vi "reward_behavior_michelle_visjitter_conswinAdapt_enticefx_TSLogFC2.vi"() -> ()   [LabVIEW 2019]
doc: "The myRIO Project template acquires acceleration data from the onboard accelerometer and displays the changes of acceleration values in a waveform chart."
uses:
  <vilib>/Analysis/Matrix/Datatypes/RealMatrix.ctl
  <vilib>/myRIO/Common/Instrument Driver Framework/myRIO v1.0/Encoder/typedefs/Encoder Signal Mode.ctl
  <vilib>/myRIO/Instrument Drivers/Onboard IO/Encoder/typedefs/Encoder Reference.ctl
  <vilib>/myRIO/Common/Instrument Driver Framework/Utilities/typedefs/myRIO Generic Hardware Reference.ctl
  <vilib>/myRIO/Common/Instrument Driver Framework/Utilities/typedefs/Hardware Version Enum.ctl
  <vilib>/myRIO/Common/Instrument Driver Framework/Utilities/typedefs/myRIO v1.0 Reference.ctl
  <vilib>/myRIO/Common/Instrument Driver Framework/Utilities/typedefs/Generic FPGA Reference.ctl
  <vilib>/myRIO/Common/Instrument Driver Framework/myRIO v1.0/Encoder/typedefs/Encoder Channels Enum.ctl
  <vilib>/myRIO/Common/Instrument Driver Framework/myRIO v1.0/Encoder/typedefs/Encoder Configuration v1.0.ctl
  <vilib>/userdefined/High Color/nirio_resource_hc.ctl
  <vilib>/myRIO/Instrument Drivers/Onboard IO/DIO/typedefs/DIO Reference.ctl
  <vilib>/myRIO/Common/Instrument Driver Framework/myRIO v1.0/DIO/typedefs/DIO Channels List.ctl
  <vilib>/myRIO/Common/Instrument Driver Framework/myRIO v1.0/DIO/typedefs/DIO Channels Enum.ctl
  <vilib>/myRIO/Common/Instrument Driver Framework/Utilities/vis/Is FPGA Ref Available.vi
  <vilib>/myRIO/Common/Instrument Driver Framework/myRIO v1.0/Encoder/vis/myRIO v1.1 Open Encoder.vi
  <vilib>/myRIO/Instrument Drivers/Onboard IO/Encoder/vis/Read.vi
  <vilib>/myRIO/Common/Instrument Driver Framework/myRIO v1.0/DIO/vis/myRIO v1.1 Open DIO.vi
  <vilib>/myRIO/Instrument Drivers/Onboard IO/DIO/vis/Write.vi
  <vilib>/myRIO/Instrument Drivers/Onboard IO/DIO/vis/Read.vi
  <vilib>/myRIO/Common/Instrument Driver Framework/Utilities/vis/Validate Channels.vi
  <vilib>/myRIO/Common/Instrument Driver Framework/myRIO v1.0/Encoder/vis/myRIO v1.0 Reserve Encoder.vi
  <vilib>/myRIO/Common/Instrument Driver Framework/myRIO v1.0/DIO/vis/myRIO v1.0 Reserve DIO.vi
  <vilib>/myRIO/Common/Instrument Driver Framework/myRIO v1.0/Encoder/vis/myRIO v1.0 Build MUX Configuration Encoder.vi
  <vilib>/myRIO/Common/Instrument Driver Framework/myRIO v1.0/Resource Manager/vis/myRIO v1.0 Reserve Channel List.vi
  <vilib>/myRIO/Common/Instrument Driver Framework/myRIO v1.0/DIO/vis/myRIO v1.0 Build MUX Configuration DIO.vi
  <vilib>/myRIO/Common/Instrument Driver Framework/myRIO v1.0/Resource Manager/vis/myRIO v1.0 Create Configuration List.vi
  <vilib>/myRIO/Common/Instrument Driver Framework/myRIO v1.0/Resource Manager/vis/myRIO v1.0 Reserve Channel.vi
  <vilib>/myRIO/Common/Instrument Driver Framework/myRIO v1.0/Resource Manager/vis/myRIO v1.0 Unreserve Channel.vi
  <vilib>/myRIO/Common/Instrument Driver Framework/myRIO v1.0/Resource Manager/vis/myRIO v1.0 Build Mutex Name.vi
  <vilib>/Utility/VariantDataType/GetNumericInfo.vi
  <vilib>/Utility/error.llb/Error Cluster From Error Code.vi
  <vilib>/myRIO/Common/Instrument Driver Framework/myRIO v1.0/myRIO v1.1 Open.vi
  <vilib>/myRIO/Common/Instrument Driver Framework/Utilities/vis/IO Manager.vi
  <vilib>/myRIO/Common/Instrument Driver Framework/Utilities/vis/Configuration Manager.vi
  <vilib>/myRIO/Common/Instrument Driver Framework/myRIO v1.0/Resource Manager/vis/myRIO v1.0 Configure IO.vi
  <vilib>/myRIO/Common/Instrument Driver Framework/myRIO v1.0/myRIO v1.0 Close.vi
  <vilib>/myRIO/Common/Instrument Driver Framework/myRIO v1.0/Encoder/vis/myRIO v1.0 Configure Encoder.vi
  <vilib>/myRIO/Common/Instrument Driver Framework/myRIO v1.0/Encoder/vis/myRIO v1.0 Read Encoder.vi
  <vilib>/myRIO/Common/Instrument Driver Framework/myRIO v1.0/DIO/vis/myRIO v1.0 Read DIO.vi
  <vilib>/myRIO/Common/Instrument Driver Framework/myRIO v1.0/DIO/vis/myRIO v1.0 Write DIO.vi
  <vilib>/myRIO/Express VI/Onboard IO/Encoder/Encoder Express VI.xnode
  <vilib>/myRIO/Instrument Drivers/Onboard IO/Encoder/vis/myRIO Encoder Open.xnode
  <vilib>/myRIO/Express VI/Onboard IO/DI/DI Express VI.xnode
  <vilib>/myRIO/Instrument Drivers/Onboard IO/DIO/vis/myRIO DIO Open.xnode
  <vilib>/myRIO/Express VI/Onboard IO/DO/DO Express VI.xnode
  <vilib>/myRIO/Instrument Drivers/Onboard IO/Encoder/Encoder.lvlib
  <vilib>/myRIO/Instrument Drivers/Onboard IO/DIO/DIO.lvlib
  <vilib>/Analysis/Matrix/NI_Matrix.lvlib
panel:
  out "EntTS":dbl[][](array[numeric])
  out "TimeLag":dbl
  out "Lag2":dbl
  out "TestTime":dbl
  out "RewTS":dbl[][](array[numeric])
  out "ConsTS":dbl[][](array[numeric])
  out "LickTS":dbl[][](array[numeric])
  out "ContrastChoice":dbl
  out "Its":i32
  out "BurstCriteria":dbl
  out "LickBurst 2":bool
  out "LickBurst":bool
  out "Enticements":i32
  in  "Entice":bool
  out "Misses":i32
  out "GoAhead":bool
  out "TimeOutDuration":i32
  out "ActiveTime":dbl
  out "ConsumptionGo":bool=TRUE
  out "Consumption_Period":i32
  out "Watch_Display":bool=TRUE
  in  "Give reward":bool
  out "Timings":dbl[](array[numeric])
  out "ISI":dbl
  out "ISI start time":dbl
  out "Time_out":bool=TRUE
  out "Time since lick":dbl
  out "Time of last lick":dbl
  out "Rewarded trials":dbl[](array[numeric])
  out "Rewards":u16
  out "Active Trial":bool
  out "Array temp2":T1
  out "Stimuli Loaded":bool
  out "Stim_ID":dbl[](array[numeric])
  out "Reward_mat":dbl[](array[numeric])
  out "Reward":bool=TRUE
  out "Frame clock":i32
  out "Licks":u32
  out "Lick":bool
  out "Time":dbl
  out "Stop":bool
  in  "Frames to collect":u32
  out "Overflow?":bool
  out "Counter Value":i32
  out "Velocity":dbl
  out "Velocity Plot":dbl[](graph)
  out "Velocity array":dbl[](array[numeric])
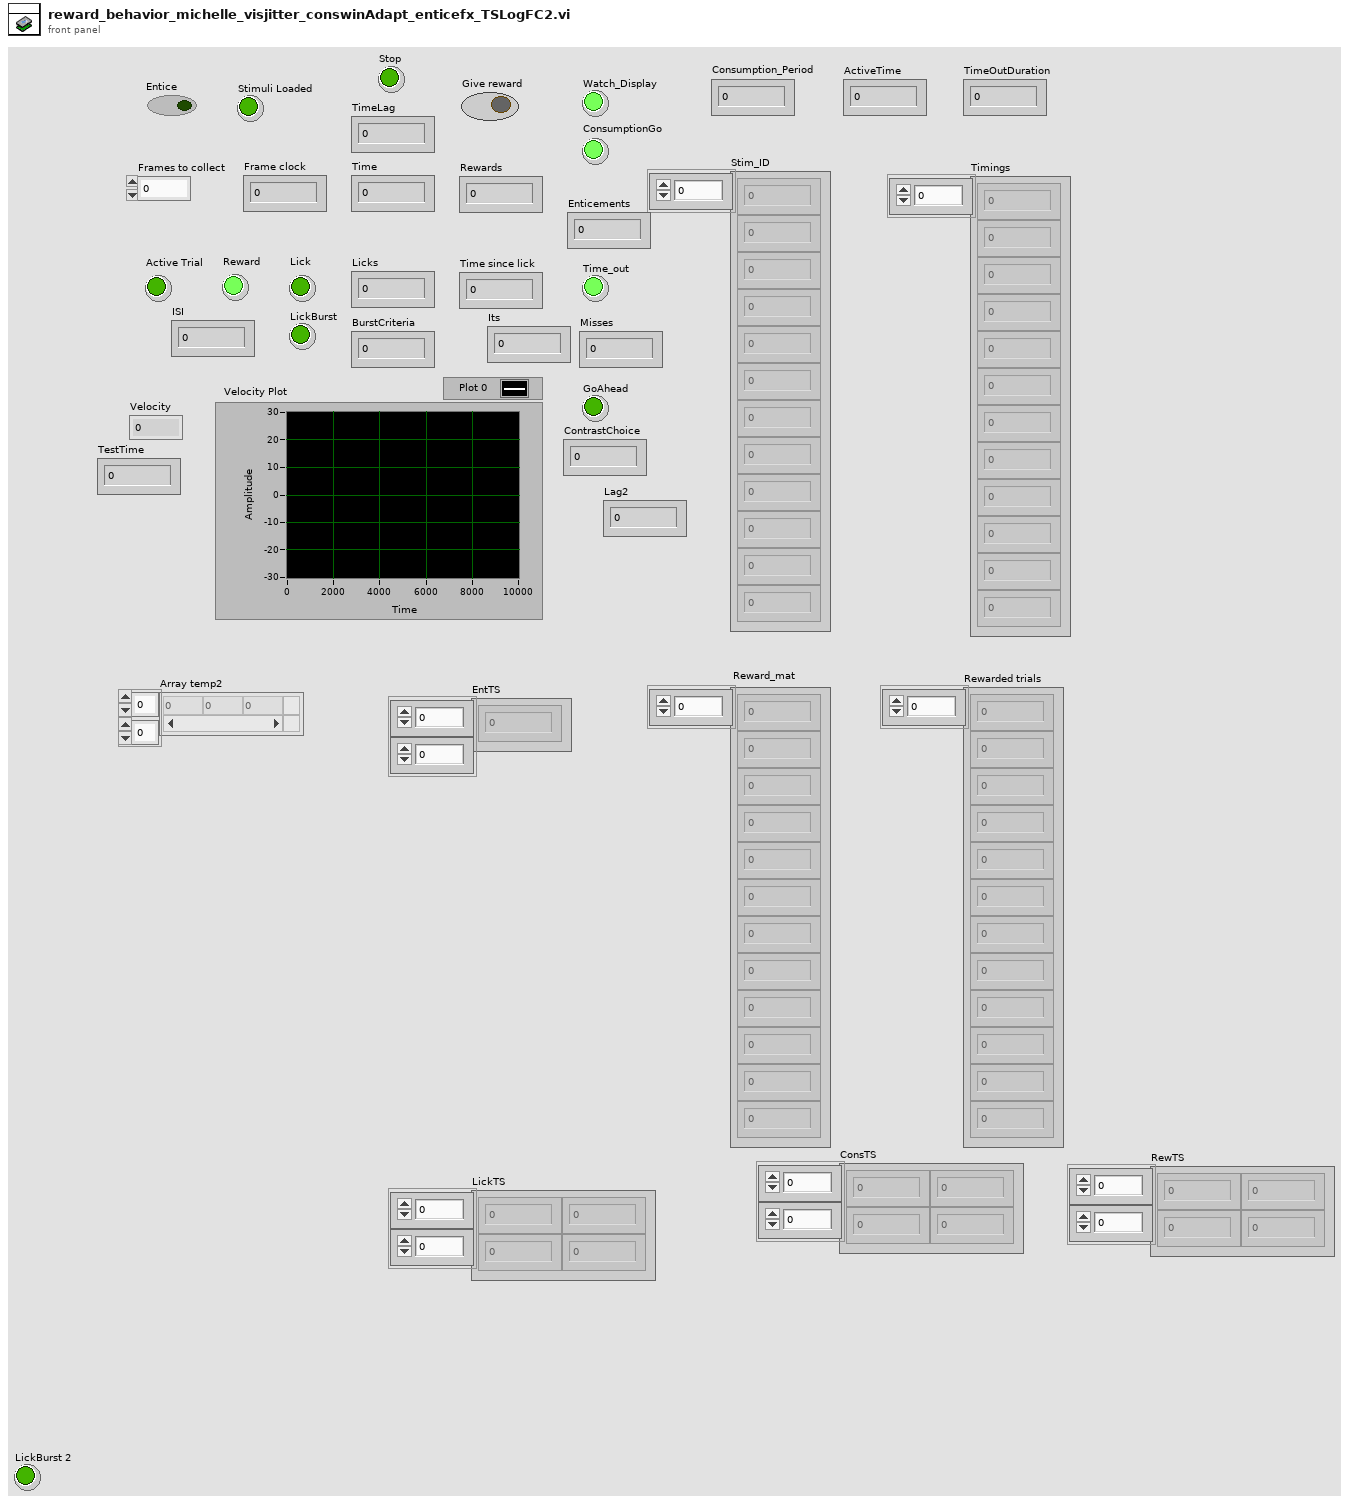
[diagram p1: front panel]
types:
  T1 = typedef "NI_Matrix.lvlib/RealMatrix.ctl" = dbl[][]
  T2 = typedef "Encoder.lvlib/Encoder Reference.ctl" = cluster{"myRIO Reference":T3, "Encoder Channels Enum":T7}
  T3 = typedef "myRIO Generic Hardware Reference.ctl" = cluster{"myRIO Model":T4, "myRIO Hardware Reference":T5}
  T4 = typedef "Hardware Version Enum.ctl" = enum16{"Unknown", "myRIO-1900", "myRIO-1950", "roboRIO", "NI ELVIS RIO CM", "ELVIS III"}
  T5 = typedef "myRIO v1.0 Reference.ctl" = cluster{"Generic FPGA Reference":T6, "Allow multiple opens":bool}
  T6 = typedef "Generic FPGA Reference.ctl" = refnum<k20>
  T7 = typedef "Encoder Channels Enum.ctl" = enum16{"Not Connected", "C/ENC0", "C/ENC1", "A/ENC", "A/ENC0", "A/ENC1", "A/ENC2", "A/ENC3", "A/ENC4", "A/ENC5", "A/ENC6", "A/ENC7", "A/ENC8", "A/ENC9", "B/ENC", "B/ENC0", "B/ENC1", "B/ENC2", "B/ENC3", "B/ENC4", "B/ENC5", "B/ENC6", "B/ENC7", "B/ENC8", "B/ENC9", "DIO/ENC0", "DIO/ENC1", "DIO/ENC2", "DIO/ENC3", "DIO/ENC4"}
  T8 = typedef "Encoder Signal Mode.ctl" = enum16{"Quadrature phase signal", "Step and direction signal"}
  T9 = typedef "nirio_resource_hc.ctl" = tag
  T10 = typedef "DIO.lvlib/DIO Reference.ctl" = cluster{"myRIO Reference":T3, "DIO Channels List":T11}
  T11 = typedef "DIO Channels List.ctl" = T12[]
  T12 = typedef "DIO Channels Enum.ctl" = enum16{"Not Connected", "C/DIO0", "C/DIO1", "C/DIO2", "C/DIO3", "C/DIO4", "C/DIO5", "C/DIO6", "C/DIO7", "A/DIO0", "A/DIO1", "A/DIO2", "A/DIO3", "A/DIO4", "A/DIO5", "A/DIO6", "A/DIO7", "A/DIO8", "A/DIO9", "A/DIO10", "A/DIO11", "A/DIO12", "A/DIO13", "A/DIO14", "A/DIO15", "A/DIO16", "A/DIO17", "A/DIO18", "A/DIO19", "B/DIO0", "B/DIO1", "B/DIO2", "B/DIO3", "B/DIO4", "B/DIO5", "B/DIO6", "B/DIO7", "B/DIO8", "B/DIO9", "B/DIO10", "B/DIO11", "B/DIO12", "B/DIO13", "B/DIO14", "B/DIO15", "B/DIO16", "B/DIO17", "B/DIO18", "B/DIO19", "LED0", "LED1", "LED2", "LED3", "Button0", "DIO/DIO0", "DIO/DIO1", "DIO/DIO2", "DIO/DIO3", "DIO/DIO4", "DIO/DIO5", "DIO/DIO6", "DIO/DIO7", "DIO/DIO8", "DIO/DIO9", "SPI/CS0", "SPI/CS1", "SPI/CS2", "SPI/CS3", "LED RADIO (Green)", "LED RADIO (Red)", "LED COMM (Green)", "LED COMM (Red)", "LED MODE (Green)", "LED MODE (Red)"}
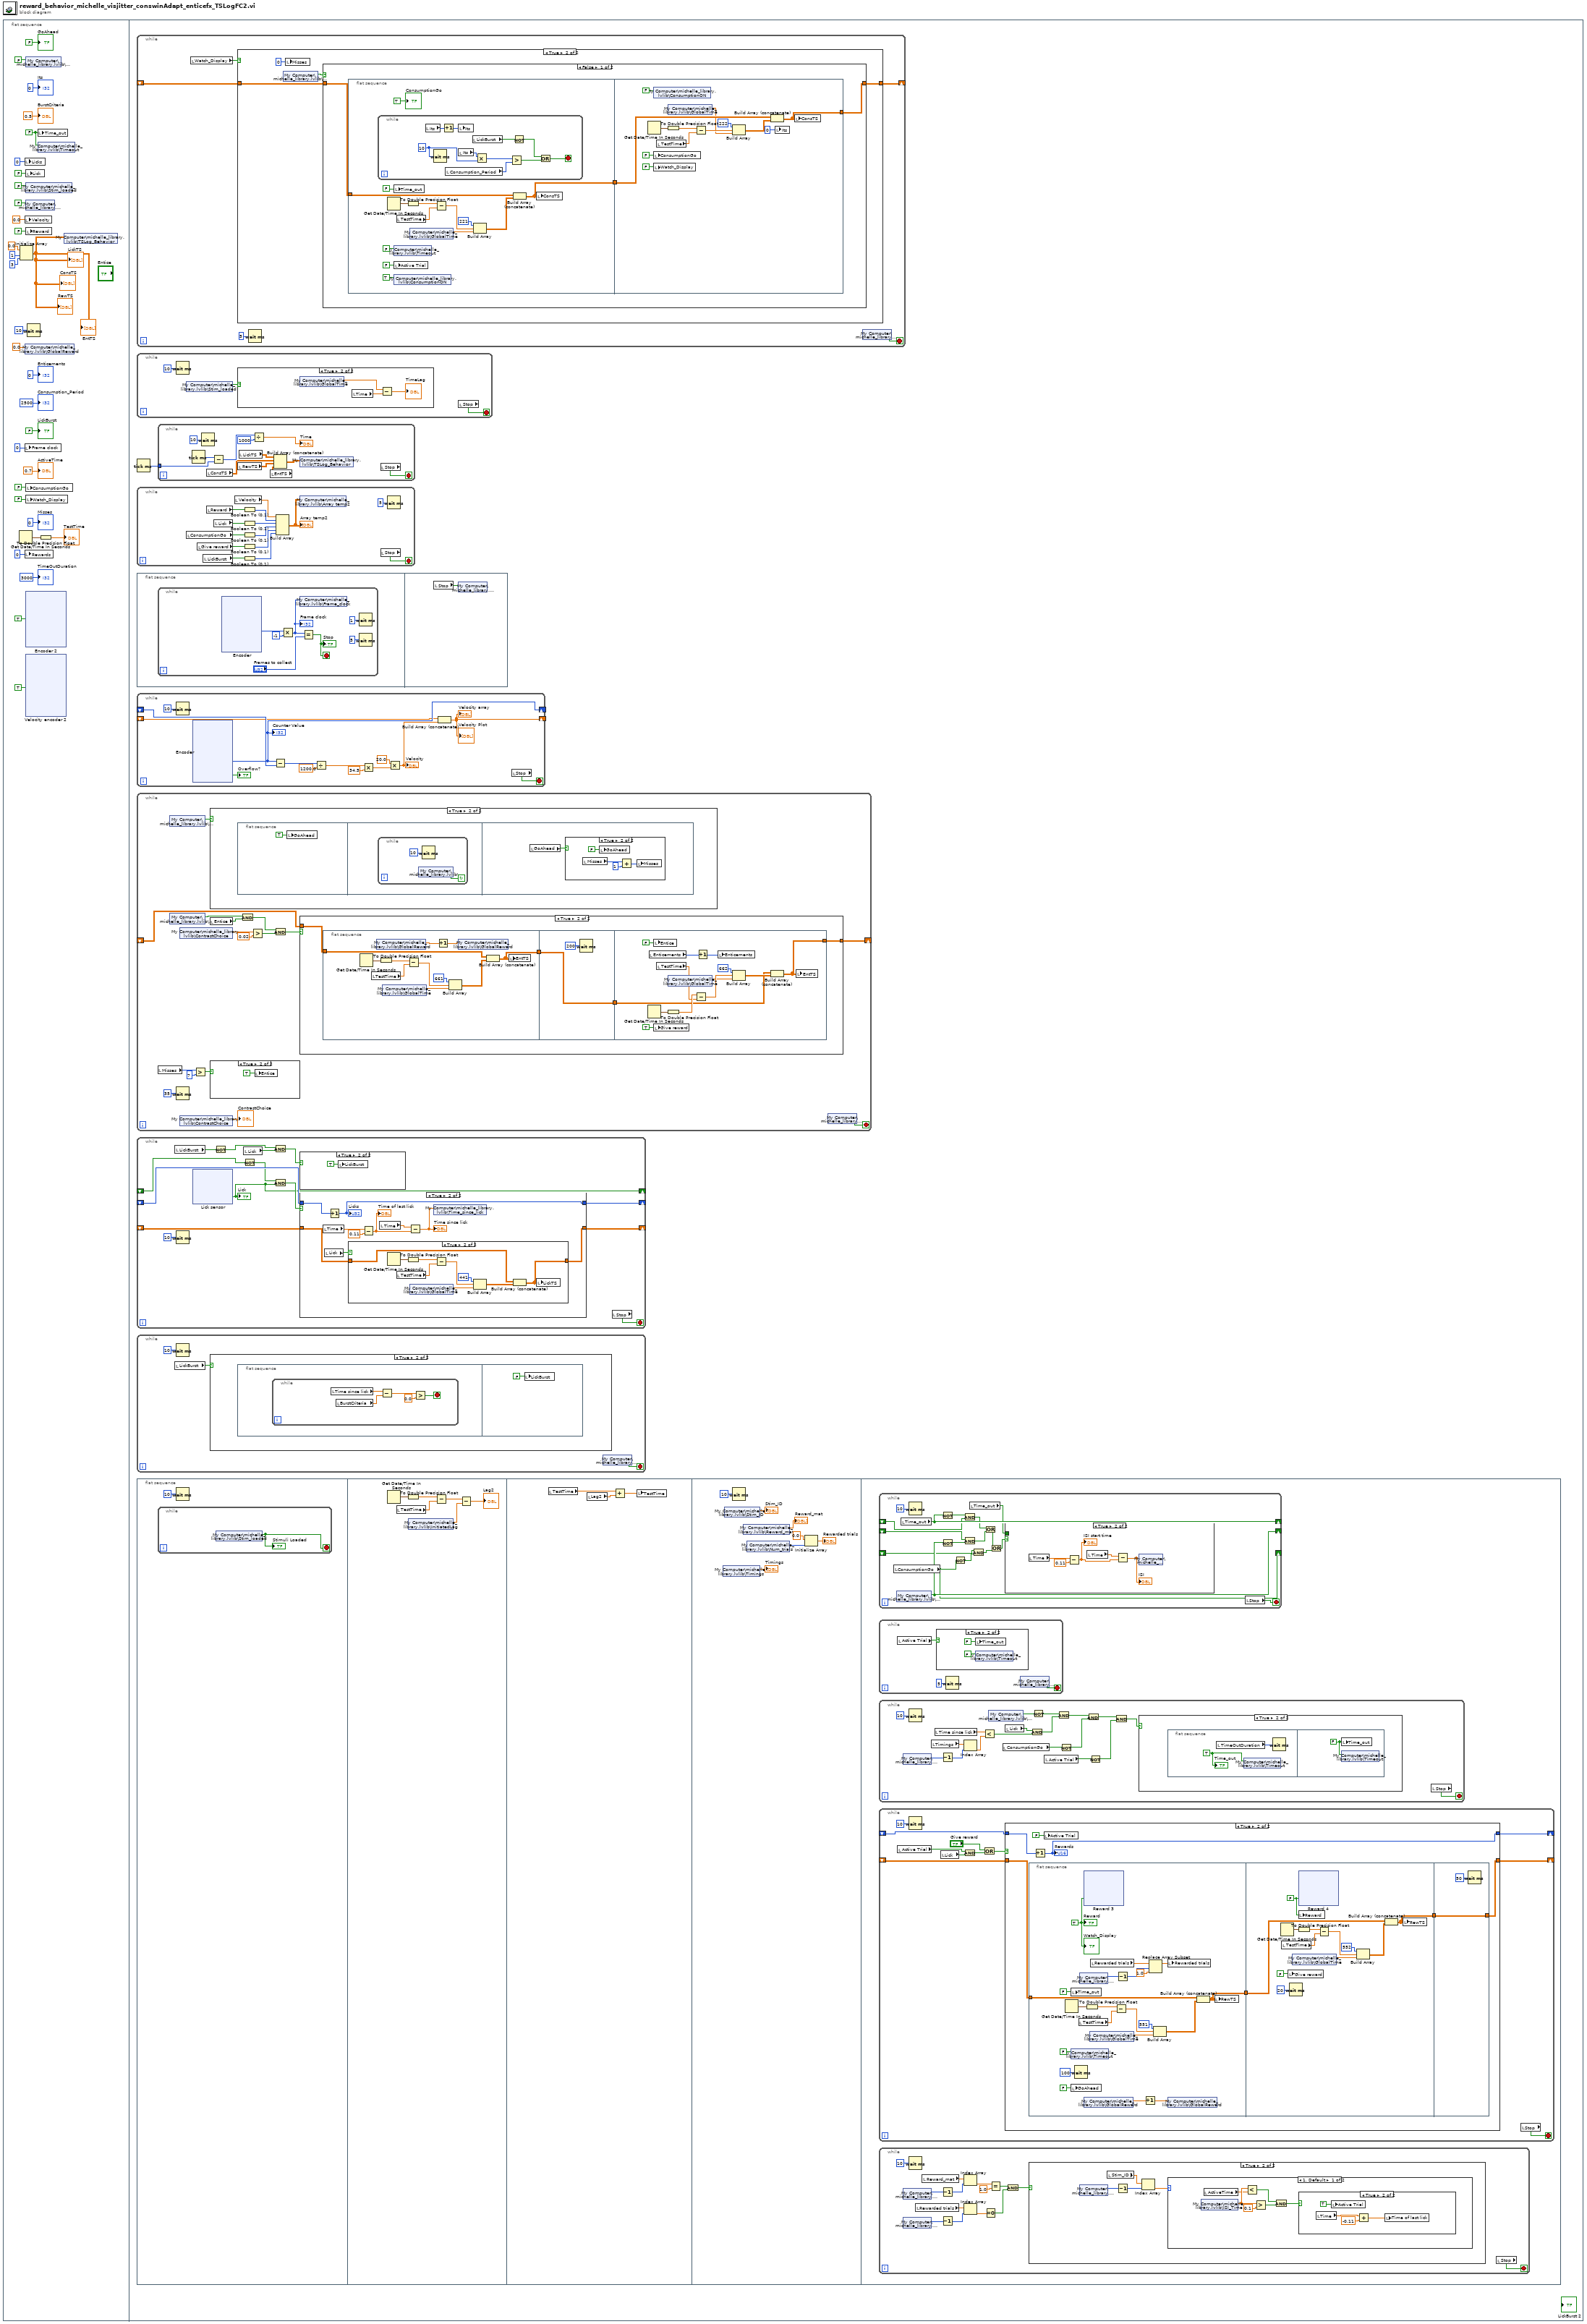
[diagram p0: block diagram]
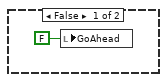
[diagram p6: hidden frame]
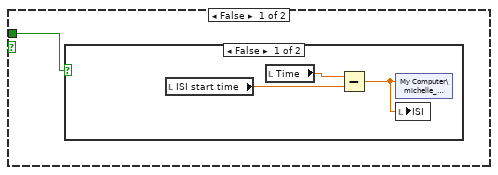
[diagram p12: hidden frame]
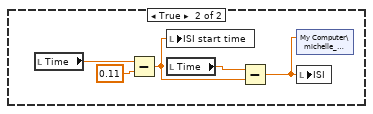
[diagram p13: hidden frame]
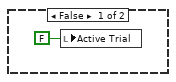
[diagram p14: hidden frame]
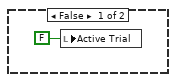
[diagram p15: hidden frame]
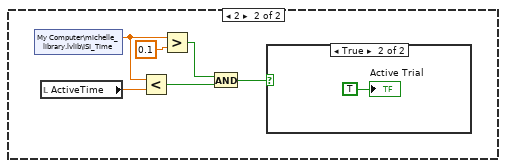
[diagram p16: hidden frame]
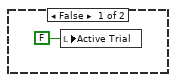
[diagram p17: hidden frame]
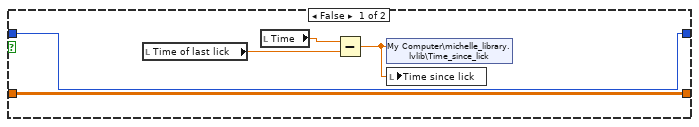
[diagram p20: hidden frame]
diagram:
  n1 = flat-sequence {
    frame #0 {
      w19 = FALSE ("Time_out")
      n2 = Get Date/Time In Seconds() -> (seconds since 1Jan1904=w3:timestamp)
      n3 = Initialize Array(0.0, 1, 3) -> (w1:dbl[][])
      "LickTS" <- w1
      "ConsTS" <- w1
      "RewTS" <- w1
      "EntTS" <- w1
      n4 = local write "Licks"(u32 0 ("Licks")) -> ()
      n5 = local write "Velocity"(0.0 ("Velocity")) -> ()
      n6 = shared-variable "My Computer\\michelle_library.lvlib\\GlobalReward"(0.0) -> ()  [unwired: 1 in, 1 out]
      n7 = local write "Frame clock"(u32 0 ("Frames")) -> ()
      n8 = local write "Rewards"(u16 0 ("Rewards")) -> ()
      n9 = shared-variable "My Computer\\michelle_library.lvlib\\Display"(FALSE ("Display")) -> ()  [unwired: 1 in, 1 out]
      n10 = local write "Lick"(FALSE ("Lick")) -> ()
      n11 = shared-variable "My Computer\\michelle_library.lvlib\\Stim_loaded"(FALSE ("Stim_loaded")) -> ()  [unwired: 1 in, 1 out]
      n12 = shared-variable "My Computer\\michelle_library.lvlib\\Stop"(FALSE ("Stop")) -> ()  [unwired: 1 in, 1 out]
      n13 = local write "Reward"(FALSE ("Give reward")) -> ()
      n14 = local write "ConsumptionGo"(FALSE ("ConsumptionGo")) -> ()
      n15 = local write "Watch_Display"(FALSE ("Watch_Display")) -> ()
      n16 = xnode "Encoder 2"("Reset Counter"=TRUE) -> ()  [unwired: 1 in, 4 out]
      n17 = xnode "Velocity encoder 2"("Reset Counter"=TRUE) -> ()  [unwired: 1 in, 4 out]
      n18 = Wait (ms)(milliseconds to wait=u32 10) -> ()  [unwired: 1 out]
      n19 = local write "Time_out"(w19) -> ()
      n20 = shared-variable "My Computer\\michelle_library.lvlib\\Timeout"(w19) -> ()  [unwired: 1 in, 1 out]
      n21 = To Double Precision Float(number=w3) -> (double precision float=→"TestTime":dbl)
      n22 = shared-variable "My Computer\\michelle_library.lvlib\\TSLog_Behavior"(w1) -> ()  [unwired: 1 in, 1 out]
      "Consumption_Period" <- 2500
      "ActiveTime" <- 0.7
      "TimeOutDuration" <- 3000
      "GoAhead" <- FALSE
      "Misses" <- 0
      "Enticements" <- 0
      "LickBurst" <- FALSE
      "BurstCriteria" <- 0.5
      "Its" <- 0
    }
    frame #1 {
      n23 = while {
        shift-right: [w197] -> _
        shift-left: _ -> [w198]
        stop <- w201 stop-if-true
        n24 = local read "Watch_Display"() -> (w200:bool)
        n25 = case shown="True" w200 {
          tunnel: w198 -> [w202 w204]
          tunnel: [w202 w203] -> w197
          frame False {
          }
          frame True {
            n26 = shared-variable "My Computer\\michelle_library.lvlib\\Display"() -> (w206:bool)  [unwired: 1 in, 1 out]
            n27 = local write "Misses"(0) -> ()
            n28 = case shown="False" w206 {
              tunnel: w204 -> [w209 w247]
              tunnel: [w207 w247] -> w203
              frame False {
                n29 = flat-sequence {
                  tunnel: w209 -> [w212]
                  tunnel: [w211] -> w208
                  tunnel: w208 -> [w237]
                  tunnel: [w236] -> w207
                  frame #0 {
                    n30 = while {
                      stop <- w227 stop-if-true
                      w228 = 10
                      n31 = local read "Its"() -> (w232:i32)
                      n32 = Wait (ms)(milliseconds to wait=w228) -> ()  [unwired: 1 out]
                      n33 = Increment(x=w232) -> (x+1=w231:i32)
                      n34 = local read "Consumption_Period"() -> (w225:i32)
                      n35 = local write "Its"(w231) -> ()
                      n36 = local read "Its"() -> (w229:i32)
                      n37 = local read "LickBurst"() -> (w233:bool)
                      n38 = Multiply(x=w229, y=w228) -> (x*y=w226:i32)
                      n39 = Greater?(x=w226, y=w225) -> (0:w224:bool)
                      n40 = Not(x=w233) -> (.not. x?=w230:bool)
                      n41 = Or(x=w230, y=w224) -> (x .or. y?=w227:bool)
                    }
                    n42 = Get Date/Time In Seconds() -> (seconds since 1Jan1904=w217:timestamp)
                    n43 = local write "Time_out"(FALSE) -> ()
                    n44 = shared-variable "My Computer\\michelle_library.lvlib\\Timeout"(FALSE) -> ()  [unwired: 1 in, 1 out]
                    n45 = local write "Active Trial"(FALSE) -> ()
                    n46 = shared-variable "My Computer\\michelle_library.lvlib\\ConsumptionON"(TRUE) -> ()  [unwired: 1 in, 1 out]
                    n47 = local read "TestTime"() -> (w214:dbl)
                    n48 = To Double Precision Float(number=w217) -> (double precision float=w215:dbl)
                    n49 = shared-variable "My Computer\\michelle_library.lvlib\\GlobalTime"() -> (w210:dbl)  [unwired: 1 in, 1 out]
                    n50 = Subtract(x=w215, y=w214) -> (x-y=w218:dbl)
                    n51 = Build Array(221, w218, w210) -> (w213:T1)
                    n52 = Build Array (concatenate) ("Build Matrix")(w212, w213) -> (w211:T1)
                    n53 = local write "ConsTS"(w211) -> ()
                    "ConsumptionGo" <- TRUE
                  }
                  frame #1 {
                    n54 = Get Date/Time In Seconds() -> (seconds since 1Jan1904=w241:timestamp)
                    n55 = shared-variable "My Computer\\michelle_library.lvlib\\ConsumptionON"(FALSE) -> ()  [unwired: 1 in, 1 out]
                    n56 = local write "ConsumptionGo"(FALSE ("ConsumptionGo")) -> ()
                    n57 = local write "Watch_Display"(FALSE ("Watch_Display")) -> ()
                    n58 = local read "TestTime"() -> (w238:dbl)
                    n59 = To Double Precision Float(number=w241) -> (double precision float=w239:dbl)
                    n60 = shared-variable "My Computer\\michelle_library.lvlib\\GlobalTime"() -> (w234:dbl)  [unwired: 1 in, 1 out]
                    n61 = Subtract(x=w239, y=w238) -> (x-y=w242:dbl)
                    n62 = Build Array(222, w242, w234) -> (w235:T1)
                    n63 = Build Array (concatenate) ("Build Matrix")(w237, w235) -> (w236:T1)
                    n64 = local write "Its"(0) -> ()
                    n65 = local write "ConsTS"(w236) -> ()
                  }
                }
              }
              frame True {
              }
            }
          }
        }
        n66 = Wait (ms)(milliseconds to wait=u32 5) -> ()  [unwired: 1 out]
        n67 = shared-variable "My Computer\\michelle_library.lvlib\\Stop"() -> (w201:bool)  [unwired: 1 in, 1 out]
      }
      n68 = while {
        stop <- w126 stop-if-true
        n69 = Wait (ms)(milliseconds to wait=u32 10) -> ()  [unwired: 1 out]
        n70 = shared-variable "My Computer\\michelle_library.lvlib\\Stim_loaded"() -> (w127:bool)  [unwired: 1 in, 1 out]
        n71 = case shown="True" w127 {
          frame False {
          }
          frame True {
            n72 = shared-variable "My Computer\\michelle_library.lvlib\\GlobalTime"() -> (w128:dbl)  [unwired: 1 in, 1 out]
            n73 = local read "Time"() -> (w129:dbl)
            n74 = Subtract(x=w128, y=w129) -> (x-y=→"TimeLag":dbl)
          }
        }
        n75 = local read "Stop"() -> (w126:bool)
      }
      n76 = Tick Count (ms)() -> (millisecond timer value=w124:u32)
      n77 = while {
        stop <- w255 stop-if-true
        n78 = local read "ConsumptionGo"() -> (w253:bool)
        n79 = local read "Give reward"() -> (w252:bool)
        n80 = local read "LickBurst"() -> (w249:bool)
        n81 = local read "Reward"() -> (w260:bool)
        n82 = local read "Lick"() -> (w261:bool)
        n83 = local read "Velocity"() -> (w259:dbl)
        n84 = Boolean To (0,1)(Boolean=w260) -> (0, 1=w258:i16)
        n85 = Boolean To (0,1)(Boolean=w261) -> (0, 1=w257:i16)
        n86 = Boolean To (0,1)(Boolean=w253) -> (0, 1=w251:i16)
        n87 = Boolean To (0,1)(Boolean=w252) -> (0, 1=w250:i16)
        n88 = Boolean To (0,1)(Boolean=w249) -> (0, 1=w248:i16)
        n89 = Build Array(w259, w258, w257, w251, w250, w248) -> (w254:T1)
        "Array temp2" <- w254
        n90 = shared-variable "My Computer\\michelle_library.lvlib\\Array temp2"(w254) -> ()  [unwired: 1 in, 1 out]
        n91 = local read "Stop"() -> (w255:bool)
        n92 = Wait (ms)(milliseconds to wait=u32 5) -> ()  [unwired: 1 out]
      }
      n93 = flat-sequence {
        frame #0 {
          n94 = while {
            stop <- w502 stop-if-true
            n95 = xnode "Encoder"() -> ("Counter Value"=w506:i32)  [unwired: 2 in, 3 out]
            n96 = Multiply(x=w506, y=-1) -> (x*y=w501:i32)
            "Frame clock" <- w501
            n97 = shared-variable "My Computer\\michelle_library.lvlib\\Frame_clock"(w501) -> ()  [unwired: 1 in, 1 out]
            n98 = Equal?(x=w501, y="Frames to collect") -> (x = y?=w502:bool)
            "Stop" <- w502
            n99 = Wait (ms)(milliseconds to wait=u32 1) -> ()  [unwired: 1 out]
            n100 = Wait (ms)(milliseconds to wait=u32 5) -> ()  [unwired: 1 out]
          }
        }
        frame #1 {
          n101 = local read "Stop"() -> (w554:bool)
          n102 = shared-variable "My Computer\\michelle_library.lvlib\\Stop"(w554) -> ()  [unwired: 1 in, 1 out]
        }
      }
      n103 = while {
        shift-right: [w640] -> _
        shift-left: _ -> [w641]
        shift-right: [w632] -> _
        shift-left: _ -> [w631]
        stop <- w630 stop-if-true
        n104 = Wait (ms)(milliseconds to wait=u32 10) -> ()  [unwired: 1 out]
        n105 = xnode "Encoder"() -> ("Counter Value"=w640:i32, "Overflow?"=→"Overflow?":bool)  [unwired: 2 in, 2 out]
        "Counter Value" <- w640
        n106 = Subtract(x=w640, y=w641) -> (x-y=w633:i32)
        n107 = Divide(x=w633, y=1200.0 ("600")) -> (x/y=w638:dbl)
        n108 = Multiply(x=w638, y=34.5) -> (x*y=w636:dbl)
        n109 = Multiply(x=20.0, y=w636) -> (x*y=w634:dbl)
        "Velocity" <- w634
        n110 = Build Array (concatenate)(w631, w634) -> (w632:dbl[])
        "Velocity Plot" <- w632
        "Velocity array" <- w632
        n111 = local read "Stop"() -> (w630:bool)
      }
      n112 = while {
        shift-right: [w140] -> _
        shift-left: _ -> [w141]
        stop <- w155 stop-if-true
        n113 = local read "Misses"() -> (w153:i32)
        n114 = shared-variable "My Computer\\michelle_library.lvlib\\Display"() -> (w154:bool)  [unwired: 1 in, 1 out]
        n115 = shared-variable "My Computer\\michelle_library.lvlib\\Display"() -> (w150:bool)  [unwired: 1 in, 1 out]
        n116 = Wait (ms)(milliseconds to wait=35) -> ()  [unwired: 1 out]
        n117 = shared-variable "My Computer\\michelle_library.lvlib\\ContrastChoice"() -> (w146:dbl)  [unwired: 1 in, 1 out]
        n118 = shared-variable "My Computer\\michelle_library.lvlib\\ContrastChoice"() -> (→"ContrastChoice":dbl)  [unwired: 1 in, 1 out]
        n119 = Greater?(x=w153, y=7) -> (0:w151:bool)
        n120 = case shown="True" w154 {
          frame False {
            n121 = local write "GoAhead"(FALSE) -> ()
          }
          frame True {
            n122 = flat-sequence {
              frame #0 {
                n123 = local write "GoAhead"(TRUE) -> ()
              }
              frame #1 {
                n124 = while {
                  stop <- w191 continue-if-true
                  n125 = shared-variable "My Computer\\michelle_library.lvlib\\Display"() -> (w191:bool)  [unwired: 1 in, 1 out]
                  n126 = Wait (ms)(milliseconds to wait=10) -> ()  [unwired: 1 out]
                }
              }
              frame #2 {
                n127 = local read "GoAhead"() -> (w192:bool)
                n128 = case shown="True" w192 {
                  frame False {
                  }
                  frame True {
                    n129 = local read "Misses"() -> (w196:i32)
                    n130 = local write "GoAhead"(FALSE) -> ()
                    n131 = Add(x=w196, y=1) -> (x+y=w194:i32)
                    n132 = local write "Misses"(w194) -> ()
                  }
                }
              }
            }
          }
        }
        n133 = local read "Entice"() -> (w149:bool)
        n134 = case shown="True" w151 {
          frame False {
          }
          frame True {
            n135 = local write "Entice"(TRUE) -> ()
          }
        }
        n136 = And(x=w150, y=w149) -> (x .and. y?=w147:bool)
        n137 = Greater?(x=w146, y=0.02) -> (0:w145:bool)
        n138 = And(x=w147, y=w145) -> (x .and. y?=w144:bool)
        n139 = case shown="True" w144 {
          tunnel: w141 -> [w156 w160]
          tunnel: [w156 w157] -> w140
          frame False {
          }
          frame True {
            n140 = flat-sequence {
              tunnel: w160 -> [w162]
              tunnel: [w161] -> w159
              tunnel: w159 -> [w172]
              tunnel: [w172] -> w158
              tunnel: w158 -> [w175]
              tunnel: [w174] -> w157
              frame #0 {
                n141 = Get Date/Time In Seconds() -> (seconds since 1Jan1904=w169:timestamp)
                n142 = local read "TestTime"() -> (w164:dbl)
                n143 = shared-variable "My Computer\\michelle_library.lvlib\\GlobalReward"() -> (w171:dbl)  [unwired: 1 in, 1 out]
                n144 = To Double Precision Float(number=w169) -> (double precision float=w168:dbl)
                n145 = shared-variable "My Computer\\michelle_library.lvlib\\GlobalTime"() -> (w163:dbl)  [unwired: 1 in, 1 out]
                n146 = Subtract(x=w168, y=w164) -> (x-y=w167:dbl)
                n147 = Increment(x=w171) -> (x+1=w170:dbl)
                n148 = Build Array(661, w167, w163) -> (w166:T1)
                n149 = shared-variable "My Computer\\michelle_library.lvlib\\GlobalReward"(w170) -> ()  [unwired: 1 in, 1 out]
                n150 = Build Array (concatenate) ("Build Matrix")(w162, w166) -> (w161:T1)
                n151 = local write "EntTS"(w161) -> ()
              }
              frame #1 {
                n152 = Wait (ms)(milliseconds to wait=200) -> ()  [unwired: 1 out]
              }
              frame #2 {
                n153 = Get Date/Time In Seconds() -> (seconds since 1Jan1904=w182:timestamp)
                n154 = local read "Enticements"() -> (w184:i32)
                n155 = local write "Entice"(FALSE) -> ()
                n156 = local write "Give reward"(TRUE) -> ()
                n157 = local read "TestTime"() -> (w176:dbl)
                n158 = To Double Precision Float(number=w182) -> (double precision float=w181:dbl)
                n159 = shared-variable "My Computer\\michelle_library.lvlib\\GlobalTime"() -> (w177:dbl)  [unwired: 1 in, 1 out]
                n160 = Subtract(x=w181, y=w176) -> (x-y=w180:dbl)
                n161 = Increment(x=w184) -> (x+1=w183:i32)
                n162 = local write "Enticements"(w183) -> ()
                n163 = Build Array(662, w180, w177) -> (w179:T1)
                n164 = Build Array (concatenate) ("Build Matrix")(w175, w179) -> (w174:T1)
                n165 = local write "EntTS"(w174) -> ()
              }
            }
          }
        }
        n166 = shared-variable "My Computer\\michelle_library.lvlib\\Stop"() -> (w155:bool)  [unwired: 1 in, 1 out]
      }
      n167 = while {
        shift-right: [w567] -> _
        shift-left: _ -> [w566]
        shift-right: [w561] -> _
        shift-left: _ -> [w564]
        shift-right: [w555] -> _
        shift-left: _ -> [w556]
        stop <- w565 stop-if-true
        n168 = local read "LickBurst"() -> (w558:bool)
        n169 = Wait (ms)(milliseconds to wait=u32 10) -> ()  [unwired: 1 out]
        n170 = xnode "Lick sensor"() -> ("C/DIO1 (DIO1)"=w561:bool)  [unwired: 1 in, 1 out]
        "Lick" <- w561
        n171 = Not(x=w558) -> (.not. x?=w557:bool)
        n172 = Not(x=w564) -> (.not. x?=w563:bool)
        n173 = local read "Lick"() -> (w559:bool)
        n174 = And(x=w557, y=w559) -> (x .and. y?=w560:bool)
        n175 = And(x=w563, y=w561) -> (x .and. y?=w562:bool)
        n176 = case shown="True" w560 {
          frame False {
          }
          frame True {
            n177 = local write "LickBurst"(TRUE) -> ()
          }
        }
        n178 = case shown="True" w562 {
          tunnel: [w574 w584] -> w567
          tunnel: w566 -> [w574 w583]
          tunnel: w556 -> [w570 w575]
          tunnel: [w570 w577] -> w555
          frame False {
            n179 = local read "Time of last lick"() -> (w572:dbl)
            n180 = local read "Time"() -> (w573:dbl)
            n181 = Subtract(x=w573, y=w572) -> (x-y=w571:dbl)
            n182 = shared-variable "My Computer\\michelle_library.lvlib\\Time_since_lick"(w571) -> ()  [unwired: 1 in, 1 out]
            n183 = local write "Time since lick"(w571) -> ()
          }
          frame True {
            n184 = local read "Time"() -> (w580:dbl)
            n185 = local read "Lick"() -> (w576:bool)
            n186 = Increment(x=w583) -> (x+1=w584:u32)
            "Licks" <- w584
            n187 = case shown="True" w576 {
              tunnel: w575 -> [w585 w590]
              tunnel: [w585 w589] -> w577
              frame False {
              }
              frame True {
                n188 = Get Date/Time In Seconds() -> (seconds since 1Jan1904=w592:timestamp)
                n189 = local read "TestTime"() -> (w587:dbl)
                n190 = To Double Precision Float(number=w592) -> (double precision float=w588:dbl)
                n191 = shared-variable "My Computer\\michelle_library.lvlib\\GlobalTime"() -> (w586:dbl)  [unwired: 1 in, 1 out]
                n192 = Subtract(x=w588, y=w587) -> (x-y=w593:dbl)
                n193 = Build Array(441, w593, w586) -> (w594:T1)
                n194 = Build Array (concatenate) ("Build Matrix")(w590, w594) -> (w589:T1)
                n195 = local write "LickTS"(w589) -> ()
              }
            }
            n196 = Subtract(x=w580, y=0.11) -> (x-y=w578:dbl)
            "Time of last lick" <- w578
            n197 = local read "Time"() -> (w582:dbl)
            n198 = Subtract(x=w582, y=w578) -> (x-y=w581:dbl)
            "Time since lick" <- w581
            n199 = shared-variable "My Computer\\michelle_library.lvlib\\Time_since_lick"(w581) -> ()  [unwired: 1 in, 1 out]
          }
        }
        n200 = local read "Stop"() -> (w565:bool)
      }
      n201 = while {
        stop <- w133 stop-if-true
        n202 = local read "LickBurst"() -> (w131:bool)
        n203 = Wait (ms)(milliseconds to wait=u32 10) -> ()  [unwired: 1 out]
        n204 = case shown="True" w131 {
          frame False {
          }
          frame True {
            n205 = flat-sequence {
              frame #0 {
                n206 = while {
                  stop <- w136 stop-if-true
                  n207 = local read "Time since lick"() -> (w137:dbl)
                  n208 = local read "BurstCriteria"() -> (w138:dbl)
                  n209 = Subtract(x=w137, y=w138) -> (x-y=w134:dbl)
                  n210 = Greater?(x=w134, y=0.0) -> (0:w136:bool)
                }
              }
              frame #1 {
                n211 = local write "LickBurst"(FALSE) -> ()
              }
            }
          }
        }
        n212 = shared-variable "My Computer\\michelle_library.lvlib\\Stop"() -> (w133:bool)  [unwired: 1 in, 1 out]
      }
      n213 = flat-sequence {
        frame #0 {
          n214 = while {
            stop <- w263 stop-if-true
            n215 = shared-variable "My Computer\\michelle_library.lvlib\\Stim_loaded"() -> (w263:bool)  [unwired: 1 in, 1 out]
            "Stimuli Loaded" <- w263
          }
          n216 = Wait (ms)(milliseconds to wait=u32 10) -> ()  [unwired: 1 out]
        }
        frame #1 {
          n217 = Get Date/Time In Seconds() -> (seconds since 1Jan1904=w269:timestamp)
          n218 = local read "TestTime"() -> (w268:dbl)
          n219 = To Double Precision Float(number=w269) -> (double precision float=w267:dbl)
          n220 = shared-variable "My Computer\\michelle_library.lvlib\\InitiatedLag"() -> (w266:dbl)  [unwired: 1 in, 1 out]
          n221 = Subtract(x=w267, y=w268) -> (x-y=w264:dbl)
          n222 = Subtract(x=w264, y=w266) -> (x-y=→"Lag2":dbl)
        }
        frame #2 {
          n223 = local read "TestTime"() -> (w270:dbl)
          n224 = local read "Lag2"() -> (w271:dbl)
          n225 = Add(x=w270, y=w271) -> (x+y=w272:dbl)
          n226 = local write "TestTime"(w272) -> ()
        }
        frame #3 {
          n227 = shared-variable "My Computer\\michelle_library.lvlib\\Timings"() -> (→"Timings":dbl[])  [unwired: 1 in, 1 out]
          n228 = shared-variable "My Computer\\michelle_library.lvlib\\Stim_ID"() -> (→"Stim_ID":dbl[])  [unwired: 1 in, 1 out]
          n229 = Wait (ms)(milliseconds to wait=u32 10) -> ()  [unwired: 1 out]
          n230 = shared-variable "My Computer\\michelle_library.lvlib\\Reward_mat"() -> (→"Reward_mat":dbl[])  [unwired: 1 in, 1 out]
          n231 = shared-variable "My Computer\\michelle_library.lvlib\\Num_trials"() -> (w276:u32)  [unwired: 1 in, 1 out]
          n232 = Initialize Array(0.0 ("element"), w276) -> (→"Rewarded trials":dbl[])
        }
        frame #4 {
          n233 = while {
            shift-right: [w322] -> _
            shift-left: _ -> [w320]
            shift-right: [w318] -> _
            shift-left: _ -> [w317]
            shift-right: [w312] -> _
            shift-left: _ -> [w310]
            stop <- w323 stop-if-true
            n234 = local read "ConsumptionGo"() -> (w312:bool)
            n235 = shared-variable "My Computer\\michelle_library.lvlib\\Display"() -> (w318:bool)  [unwired: 1 in, 1 out]
            n236 = local read "Time_out"() -> (w322:bool)
            n237 = Wait (ms)(milliseconds to wait=u32 10) -> ()  [unwired: 1 out]
            n238 = Not(x=w322) -> (.not. x?=w321:bool)
            n239 = Not(x=w318) -> (.not. x?=w316:bool)
            n240 = Not(x=w312) -> (.not. x?=w313:bool)
            n241 = And(x=w321, y=w320) -> (x .and. y?=w315:bool)
            n242 = And(x=w317, y=w316) -> (x .and. y?=w311:bool)
            n243 = local read "Time_out"() -> (w319:bool)
            n244 = And(x=w310, y=w313) -> (x .and. y?=w309:bool)
            n245 = Or(x=w315, y=w311) -> (x .or. y?=w308:bool)
            n246 = Or(x=w308, y=w309) -> (x .or. y?=w307:bool)
            n247 = case shown="True" w307 {
              tunnel: w319 -> [w324 _]
              frame False {
                n248 = case shown="False" w324 {
                  frame False {
                    n249 = local read "ISI start time"() -> (w327:dbl)
                    n250 = local read "Time"() -> (w326:dbl)
                    n251 = Subtract(x=w326, y=w327) -> (x-y=w325:dbl)
                    n252 = shared-variable "My Computer\\michelle_library.lvlib\\ISI"(w325) -> ()  [unwired: 1 in, 1 out]
                    n253 = local write "ISI"(w325) -> ()
                  }
                  frame True {
                    n254 = local read "Time"() -> (w332:dbl)
                    n255 = Subtract(x=w332, y=0.11) -> (x-y=w329:dbl)
                    n256 = local write "ISI start time"(w329) -> ()
                    n257 = local read "Time"() -> (w330:dbl)
                    n258 = Subtract(x=w330, y=w329) -> (x-y=w328:dbl)
                    n259 = shared-variable "My Computer\\michelle_library.lvlib\\ISI"(w328) -> ()  [unwired: 1 in, 1 out]
                    n260 = local write "ISI"(w328) -> ()
                  }
                }
              }
              frame True {
                n261 = local read "Time"() -> (w337:dbl)
                n262 = Subtract(x=w337, y=0.11) -> (x-y=w334:dbl)
                "ISI start time" <- w334
                n263 = local read "Time"() -> (w335:dbl)
                n264 = Subtract(x=w335, y=w334) -> (x-y=w333:dbl)
                "ISI" <- w333
                n265 = shared-variable "My Computer\\michelle_library.lvlib\\ISI"(w333) -> ()  [unwired: 1 in, 1 out]
              }
            }
            n266 = local read "Stop"() -> (w323:bool)
          }
          n267 = while {
            stop <- w282 stop-if-true
            n268 = local read "Active Trial"() -> (w281:bool)
            n269 = case shown="True" w281 {
              frame False {
              }
              frame True {
                n270 = local write "Time_out"(FALSE) -> ()
                n271 = shared-variable "My Computer\\michelle_library.lvlib\\Timeout"(FALSE) -> ()  [unwired: 1 in, 1 out]
              }
            }
            n272 = Wait (ms)(milliseconds to wait=5) -> ()  [unwired: 1 out]
            n273 = shared-variable "My Computer\\michelle_library.lvlib\\Stop"() -> (w282:bool)  [unwired: 1 in, 1 out]
          }
          n274 = while {
            stop <- w303 stop-if-true
            n275 = shared-variable "My Computer\\michelle_library.lvlib\\Trial"() -> (w293:u32)  [unwired: 1 in, 1 out]
            n276 = Wait (ms)(milliseconds to wait=u32 10) -> ()  [unwired: 1 out]
            n277 = local read "Timings"() -> (w295:dbl[])
            n278 = local read "Time since lick"() -> (w302:dbl)
            n279 = Decrement(x=w293) -> (x-1=w292:u32)
            n280 = Index Array(array=w295, index=w292) -> (element=w294:dbl)
            n281 = Less?(x=w302, y=w294) -> (x < y?=w301:bool)
            n282 = shared-variable "My Computer\\michelle_library.lvlib\\Display"() -> (w298:bool)  [unwired: 1 in, 1 out]
            n283 = local read "ConsumptionGo"() -> (w290:bool)
            n284 = local read "Lick"() -> (w300:bool)
            n285 = And(x=w300, y=w301) -> (x .and. y?=w296:bool)
            n286 = Not(x=w298) -> (.not. x?=w297:bool)
            n287 = local read "Active Trial"() -> (w285:bool)
            n288 = And(x=w297, y=w296) -> (x .and. y?=w289:bool)
            n289 = Not(x=w290) -> (.not. x?=w291:bool)
            n290 = And(x=w289, y=w291) -> (x .and. y?=w287:bool)
            n291 = Not(x=w285) -> (.not. x?=w288:bool)
            n292 = And(x=w287, y=w288) -> (x .and. y?=w286:bool)
            n293 = case shown="True" w286 {
              frame False {
              }
              frame True {
                n294 = flat-sequence {
                  frame #0 {
                    w305 = TRUE
                    n295 = local read "TimeOutDuration"() -> (w304:i32)
                    n296 = shared-variable "My Computer\\michelle_library.lvlib\\Timeout"(w305) -> ()  [unwired: 1 in, 1 out]
                    n297 = Wait (ms)(milliseconds to wait=w304) -> ()  [unwired: 1 out]
                    "Time_out" <- w305
                  }
                  frame #1 {
                    w306 = FALSE ("Timeout")
                    n298 = local write "Time_out"(w306) -> ()
                    n299 = shared-variable "My Computer\\michelle_library.lvlib\\Timeout"(w306) -> ()  [unwired: 1 in, 1 out]
                  }
                }
              }
            }
            n300 = local read "Stop"() -> (w303:bool)
          }
          n301 = while {
            shift-right: [w384] -> _
            shift-left: _ -> [w383]
            shift-right: [w376] -> _
            shift-left: _ -> [w377]
            stop <- w386 stop-if-true
            n302 = local read "Active Trial"() -> (w381:bool)
            n303 = Wait (ms)(milliseconds to wait=u32 10) -> ()  [unwired: 1 out]
            n304 = local read "Lick"() -> (w382:bool)
            n305 = And(x=w381, y=w382) -> (x .and. y?=w380:bool)
            n306 = Or(x="Give reward", y=w380) -> (x .or. y?=w379:bool)
            n307 = case shown="True" w379 {
              tunnel: [w388 w395] -> w384
              tunnel: w383 -> [w388 w394]
              tunnel: w377 -> [w387 w392]
              tunnel: [w387 w391] -> w376
              frame False {
              }
              frame True {
                n308 = flat-sequence {
                  tunnel: w392 -> [w400]
                  tunnel: [w397] -> w389
                  tunnel: [w455] -> w390
                  tunnel: w389 -> [w453]
                  tunnel: [w499] -> w391
                  tunnel: w390 -> [w499]
                  frame #0 {
                    w415 = TRUE ("C/DIO0 (DIO0)")
                    n309 = Get Date/Time In Seconds() -> (seconds since 1Jan1904=w404:timestamp)
                    n310 = local write "Time_out"(FALSE) -> ()
                    n311 = shared-variable "My Computer\\michelle_library.lvlib\\Timeout"(FALSE) -> ()  [unwired: 1 in, 1 out]
                    n312 = local write "GoAhead"(FALSE) -> ()
                    n313 = Wait (ms)(milliseconds to wait=u32 100) -> ()  [unwired: 1 out]
                    n314 = local read "TestTime"() -> (w398:dbl)
                    n315 = shared-variable "My Computer\\michelle_library.lvlib\\Trial"() -> (w414:u32)  [unwired: 1 in, 1 out]
                    n316 = xnode "Reward 3"("C/DIO0 (DIO0)"=w415) -> ()  [unwired: 1 in, 1 out]
                    n317 = shared-variable "My Computer\\michelle_library.lvlib\\GlobalReward"() -> (w406:dbl)  [unwired: 1 in, 1 out]
                    n318 = To Double Precision Float(number=w404) -> (double precision float=w403:dbl)
                    n319 = shared-variable "My Computer\\michelle_library.lvlib\\GlobalTime"() -> (w396:dbl)  [unwired: 1 in, 1 out]
                    n320 = local read "Rewarded trials"() -> (w412:dbl[])
                    n321 = Subtract(x=w403, y=w398) -> (x-y=w402:dbl)
                    n322 = Decrement(x=w414) -> (x-1=w413:u32)
                    n323 = Increment(x=w406) -> (x+1=w405:dbl)
                    n324 = Replace Array Subset(array=w412, new element=1.0 ("new element/subarray"), index=w413) -> (w410:dbl[])
                    n325 = Build Array(551, w402, w396) -> (w401:T1)
                    n326 = local write "Rewarded trials"(w410) -> ()
                    n327 = shared-variable "My Computer\\michelle_library.lvlib\\GlobalReward"(w405) -> ()  [unwired: 1 in, 1 out]
                    n328 = Build Array (concatenate) ("Build Matrix")(w400, w401) -> (w397:T1)
                    n329 = local write "RewTS"(w397) -> ()
                    "Reward" <- w415
                    "Watch_Display" <- w415
                  }
                  frame #1 {
                    w463 = FALSE ("C/DIO0 (DIO0)")
                    n330 = Get Date/Time In Seconds() -> (seconds since 1Jan1904=w460:timestamp)
                    n331 = local read "TestTime"() -> (w454:dbl)
                    n332 = local write "Give reward"(FALSE ("Give reward")) -> ()
                    n333 = Wait (ms)(milliseconds to wait=u32 20) -> ()  [unwired: 1 out]
                    n334 = shared-variable "My Computer\\michelle_library.lvlib\\GlobalTime"() -> (w452:dbl)  [unwired: 1 in, 1 out]
                    n335 = To Double Precision Float(number=w460) -> (double precision float=w459:dbl)
                    n336 = xnode "Reward 4"("C/DIO0 (DIO0)"=w463) -> ()  [unwired: 1 in, 1 out]
                    n337 = local write "Reward"(w463) -> ()
                    n338 = Subtract(x=w459, y=w454) -> (x-y=w458:dbl)
                    n339 = Build Array(552, w458, w452) -> (w456:T1)
                    n340 = Build Array (concatenate) ("Build Matrix")(w453, w456) -> (w455:T1)
                    n341 = local write "RewTS"(w455) -> ()
                  }
                  frame #2 {
                    n342 = Wait (ms)(milliseconds to wait=u32 50) -> ()  [unwired: 1 out]
                  }
                }
                n343 = Increment(x=w394) -> (x+1=w395:u16)
                "Rewards" <- w395
                n344 = local write "Active Trial"(FALSE ("Active Trial")) -> ()
              }
            }
            n345 = local read "Stop"() -> (w386:bool)
          }
          n346 = while {
            stop <- w351 stop-if-true
            n347 = shared-variable "My Computer\\michelle_library.lvlib\\Trial"() -> (w347:u32)  [unwired: 1 in, 1 out]
            n348 = shared-variable "My Computer\\michelle_library.lvlib\\Trial"() -> (w343:u32)  [unwired: 1 in, 1 out]
            n349 = Wait (ms)(milliseconds to wait=u32 10) -> ()  [unwired: 1 out]
            n350 = local read "Rewarded trials"() -> (w344:dbl[])
            n351 = local read "Reward_mat"() -> (w346:dbl[])
            n352 = Decrement(x=w347) -> (x-1=w348:u32)
            n353 = Decrement(x=w343) -> (x-1=w342:u32)
            n354 = Index Array(array=w346, index=w348) -> (element=w349:dbl)
            n355 = Index Array(array=w344, index=w342) -> (element=w341:dbl)
            n356 = Equal To 0?(x=w341) -> (x = 0?=w340:bool)
            n357 = Equal?(x=w349, y=1.0) -> (x = y?=w339:bool)
            n358 = And(x=w339, y=w340) -> (x .and. y?=w338:bool)
            n359 = case shown="True" w338 {
              frame False {
                n360 = local write "Active Trial"(FALSE ("Active_trial")) -> ()
              }
              frame True {
                n361 = shared-variable "My Computer\\michelle_library.lvlib\\Trial"() -> (w354:u32)  [unwired: 1 in, 1 out]
                n362 = local read "Stim_ID"() -> (w356:dbl[])
                n363 = Decrement(x=w354) -> (x-1=w355:u32)
                n364 = Index Array(array=w356, index=w355) -> (element=w353:dbl)
                n365 = case shown="1, Default" w353 {
                  frame 1, Default {
                    n366 = shared-variable "My Computer\\michelle_library.lvlib\\ISI_Time"() -> (w362:dbl)  [unwired: 1 in, 1 out]
                    n367 = local read "ActiveTime"() -> (w357:dbl)
                    n368 = Less?(x=w362, y=w357) -> (x < y?=w360:bool)
                    n369 = Greater?(x=w362, y=0.1) -> (0:w359:bool)
                    n370 = And(x=w360, y=w359) -> (x .and. y?=w358:bool)
                    n371 = case shown="True" w358 {
                      frame False {
                        n372 = local write "Active Trial"(FALSE ("Active Trial")) -> ()
                      }
                      frame True {
                        n373 = local read "Time"() -> (w366:dbl)
                        n374 = local write "Active Trial"(TRUE ("Active Trial")) -> ()
                        n375 = Add(x=w366, y=-0.11) -> (x+y=w364:dbl)
                        n376 = local write "Time of last lick"(w364) -> ()
                      }
                    }
                  }
                  frame 2 {
                    n377 = shared-variable "My Computer\\michelle_library.lvlib\\ISI_Time"() -> (w372:dbl)  [unwired: 1 in, 1 out]
                    n378 = local read "ActiveTime"() -> (w368:dbl)
                    n379 = Less?(x=w372, y=w368) -> (x < y?=w370:bool)
                    n380 = Greater?(x=w372, y=0.1) -> (0:w371:bool)
                    n381 = And(x=w371, y=w370) -> (x .and. y?=w369:bool)
                    n382 = case shown="True" w369 {
                      frame False {
                        n383 = local write "Active Trial"(FALSE ("Active Trial")) -> ()
                      }
                      frame True {
                        "Active Trial" <- TRUE ("Active Trial")
                      }
                    }
                  }
                }
              }
            }
            n384 = local read "Stop"() -> (w351:bool)
          }
        }
      }
      n385 = while {
        tunnel: w124 -> [w700]
        stop <- w698 stop-if-true
        n386 = Tick Count (ms)() -> (millisecond timer value=w701:u32)
        n387 = Wait (ms)(milliseconds to wait=u32 10) -> ()  [unwired: 1 out]
        n388 = local read "ConsTS"() -> (w693:dbl[][])
        n389 = Subtract(x=w701, y=w700) -> (x-y=w697:u32)
        n390 = local read "RewTS"() -> (w692:dbl[][])
        n391 = local read "LickTS"() -> (w694:dbl[][])
        n392 = Divide(x=w697, y=u32 1000) -> (x/y=→"Time":dbl)
        n393 = local read "EntTS"() -> (w690:dbl[][])
        n394 = Build Array (concatenate) ("Build Matrix")(w694, w693, w692, w690) -> (w691:T1)
        n395 = shared-variable "My Computer\\michelle_library.lvlib\\TSLog_Behavior"(w691) -> ()  [unwired: 1 in, 1 out]
        n396 = local read "Stop"() -> (w698:bool)
      }
    }
  }
